vi "Main.vi"(8 "error in (no error)":errorcluster, 11 "Process in":refnum<class "Input Process.lvclass">) -> (0 "error out":errorcluster, 3 "Process out":refnum<class "Input Process.lvclass">)   [LabVIEW 2019, in "TimingDRV Engine.lvlib" / "Input Process.lvclass"]
uses:
  Input Process.lvclass
  C:/Users/XEnderMD/Desktop/CD Project Tools/Source/Engine/Parent Classes/Process/Process.lvclass
  Parent Classes/Process/Process.lvclass
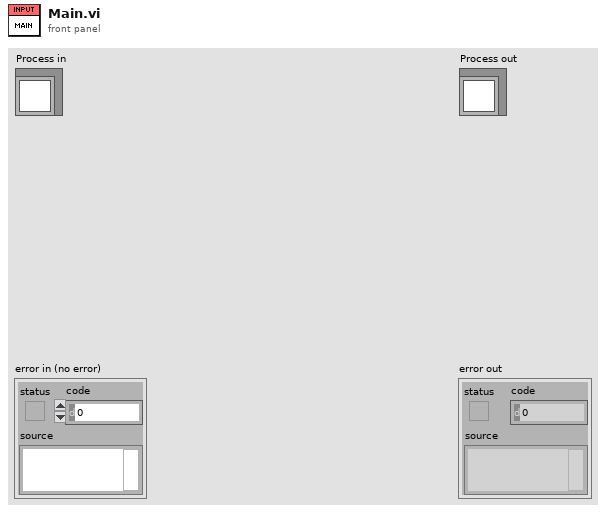
[diagram p1: front panel]
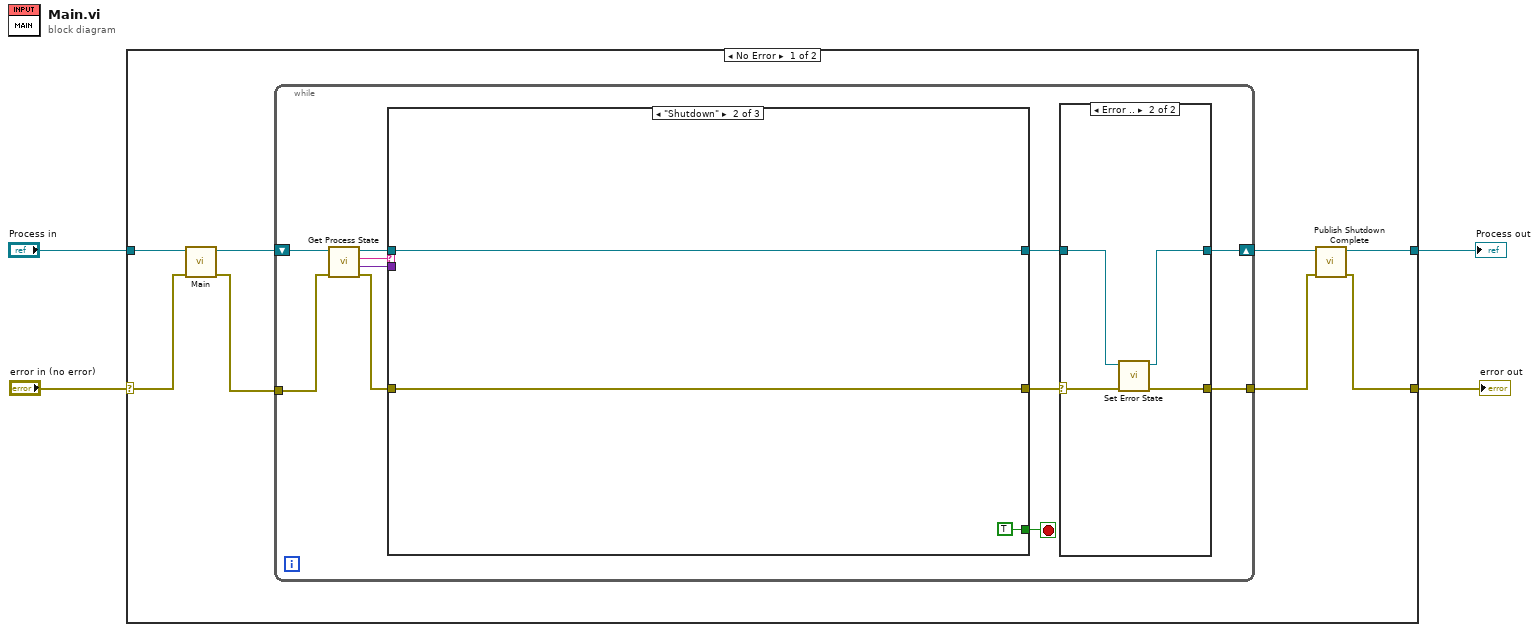
[diagram p0: block diagram]
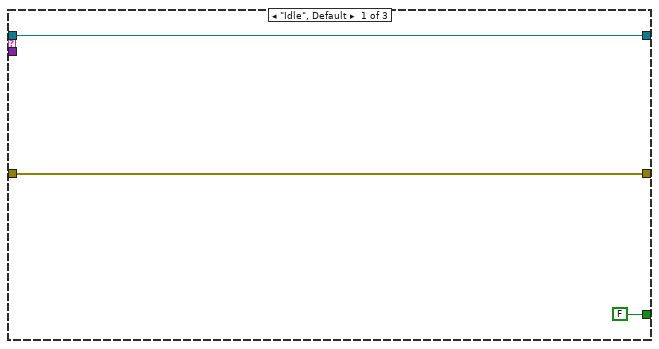
[diagram p3: hidden frame]
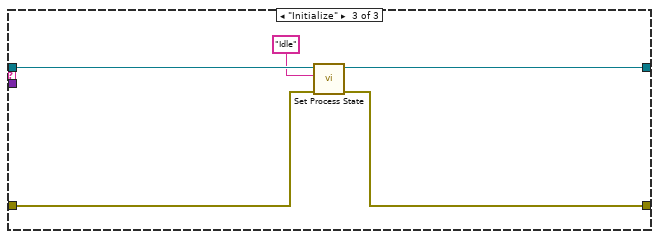
[diagram p4: hidden frame]
diagram:
  n1 = case shown="No Error" "error in (no error)" {
    selector: "error in (no error)" -> [w11 w42]
    tunnel: [w5 w42] -> w1
    tunnel: [w7 w41] -> w2
    tunnel: "Process in" -> [w12 w41]
    frame No Error {
      n2 = call-parent "Main.vi"("error in (no error)"=w11, "Process in"=w12) -> ("error out"=w9:errorcluster, "Process out"=w10:refnum<class "Input Process.lvclass">)  [unwired: 8 in]
      n3 = while {
        shift-right: [w15] -> w8
        shift-left: w10 -> [w22]
        tunnel: w9 -> [w23]
        tunnel: [w14] -> w6
        stop <- w13 stop-if-true
        n4 = call "Get Process State.vi"("error in (no error)"=w23, "Process in"=w22) -> ("error out"=w18:errorcluster, "Payload"=w19:variant, "Command"=w20:string, "Process out"=w21:refnum<class "Input Process.lvclass">)  [unwired: 6 in]
        n5 = case shown="\"Shutdown\"" w20 {
          tunnel: w21 -> [w30 w35 w40]
          tunnel: w19 -> [_ _ _]
          tunnel: w18 -> [w32 w34 w39]
          tunnel: [w30 w35 w38] -> w17
          tunnel: [w32 w34 w37] -> w16
          tunnel: [FALSE TRUE _] -> w13
          frame "Idle", Default {
          }
          frame "Shutdown" {
          }
          frame "Initialize" {
            n6 = call "Set Process State.vi"("error in (no error)"=w39, "Command"="Idle", "Process in"=w40) -> ("error out"=w37:errorcluster, "Process out"=w38:refnum<class "Input Process.lvclass">)  [unwired: 7 in]
          }
        }
        n7 = case shown="Error .." w16 {
          selector: w16 -> [w24 w29]
          tunnel: w17 -> [w25 w28]
          tunnel: [w25 w27] -> w15
          tunnel: [w24 w26] -> w14
          frame No Error {
          }
          frame Error {
            n8 = call "Set Error State.vi"("error in (no error)"=w29, "Process in"=w28) -> ("error out"=w26:errorcluster, "Process out"=w27:refnum<class "Input Process.lvclass">)  [unwired: 8 in]
          }
        }
      }
      n9 = call "Publish Shutdown Complete.vi"("error in (no error)"=w6, "Process in"=w8) -> ("error out"=w5:errorcluster, "Process out"=w7:refnum<class "Input Process.lvclass">)  [unwired: 8 in]
    }
    frame Error {
    }
  }
  "error out" <- w1
  "Process out" <- w2
